vi "Create New FIFO Instance Configuration.vi"(7 "Publisher Array in":refnum<class "CIFChannels.lvclass">[](array[class]), 10 "New FIFO Instance Config":T1 {"Custom Data" format="%.0x"}, 11 "CIFChannels.lvclass":refnum<class "CIFChannels.lvclass">) -> (2 "Flattened FIFO Config":u8[](array[numeric]), 3 "New Publisher":string)   [LabVIEW 2021, in "ChannelCommon.lvlib"]
uses:
  ChannelCommon.lvlib
  CIFChannels/CIFChannels.lvclass
  typedef/New FIFO Instance Configuration.ctl
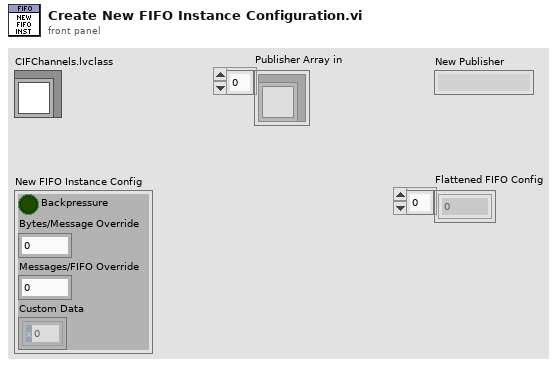
[diagram p1: front panel]
types:
  T1 = typedef "ChannelCommon.lvlib/New FIFO Instance Configuration.ctl" = cluster{"Backpressure":bool, "Bytes/Message Override":u32, "Messages/FIFO Override":u32, "Custom Data":u8[]}
  T2 = typedef "ChannelCommon.lvlib/FIFO Config.ctl" = cluster{"Max Bytes/Msg":u64, "Max Msg/FIFO":u64, "Flags":u64}
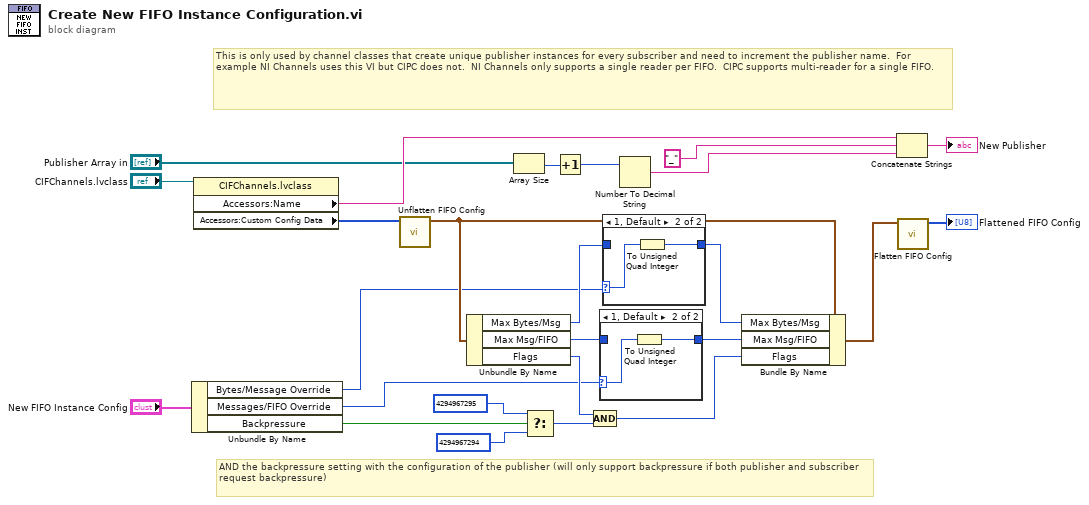
[diagram p0: block diagram]
diagram:
  # "This is only used by channel classes that create unique publisher instances for every subscriber and need to increment the publisher name.  For example NI Channels uses this VI but CIPC does not.  NI Channels only supports a single reader per FIFO.  CIPC supports multi-reader for a single FIFO."
  # "AND the backpressure setting with the configuration of the publisher (will only support backpressure if both publisher and subscriber request backpressure)"
  n1 = Unbundle By Name("New FIFO Instance Config") -> ("Bytes/Message Override"=w2:u32, "Messages/FIFO Override"=w17:u32, "Backpressure"=w22:bool)
  n2 = property class="CIFChannels.lvclass"(reference="CIFChannels.lvclass") -> ("Accessors:Name"=w25:string, "Accessors:Custom Config Data"=w23:u8[])  [unwired: 1 in, 2 out]
  n3 = call "Unflatten FIFO Config.vi"("Flattened Data in"=w23) -> ("FIFO Config out"=w15:T2)  [unwired: 9 in, 1 out]
  n4 = Unbundle By Name(w15) -> ("Max Bytes/Msg"=w3:u64, "Max Msg/FIFO"=w16:u64, "Flags"=w18:u64)
  n5 = Array Size(array="Publisher Array in") -> (size(s)=w6:i32)
  n6 = Select(t=u64 4294967295 ("Flags"), s=w22, f=u64 4294967294 ("Flags")) -> (s? t:f=w19:u64)
  n7 = Increment(x=w6) -> (x+1=w4:i32)
  n8 = Compound Arithmetic op=AND(w18, w19) -> (w13:u64)
  n9 = case shown="1, Default" w17 {
    selector: w17 -> [_ w28]
    tunnel: w16 -> [w26 _]
    tunnel: [w26 w27] -> w14
    frame 0 {
    }
    frame 1, Default {
      n10 = To Unsigned Quad Integer(1:w28) -> (0:w27:u64)
    }
  }
  n11 = case shown="1, Default" w2 {
    selector: w2 -> [_ w31]
    tunnel: w3 -> [w29 _]
    tunnel: [w29 w30] -> w1
    frame 0 {
    }
    frame 1, Default {
      n12 = To Unsigned Quad Integer(1:w31) -> (0:w30:u64)
    }
  }
  n13 = Number To Decimal String(number=w4) -> (decimal integer string=w9:string)  [unwired: 1 in]
  n14 = Bundle By Name(cluster=w15, "Max Bytes/Msg"=w1, "Max Msg/FIFO"=w14, "Flags"=w13) -> (w12:T2)
  n15 = Concatenate Strings(w25, "_", w9) -> (→"New Publisher":string)
  n16 = call "Flatten FIFO Config.vi"("FIFO Config in"=w12) -> ("Flattened FIFO Config"=→"Flattened FIFO Config":u8[])  [unwired: 10 in]
